vi "simulate or real stream sensorion data (subVI).vi"(0 "logfile refnum":refnum<file>, 1 "VISA resource name (COM3)":refnum<visa-resource-name>="COM3", 2 "stop channel":T2, 3 "abort? (F)":bool, 7 "simulate?":bool, 11 "error in (no error)":errorcluster) -> (4 "logfile refnum out":refnum<file>, 8 "sensor data cluster \nstream channel":T1, 15 "error out":errorcluster)   [LabVIEW 2021]
uses:
  <extravilib>/ChannelInstances/Tag-bool/))Channel.ctl
  <extravilib>/ChannelInstances/Stream-t'sensirion_data_with_time.ctl'/)Channel.ctl
  type-defs/sensirion_data_with_time.ctl
  controls/sensirion_flow_sensor_data.ctl
  <extravilib>/ChannelInstances/Tag-bool/Write With Abort.vi
  <extravilib>/ChannelInstances/Tag-bool/Read With Abort.vi
  <extravilib>/ChannelInstances/Stream-t'sensirion_data_with_time.ctl'/Read With Abort.vi
  <extravilib>/ChannelInstances/Stream-t'sensirion_data_with_time.ctl'/Write With Abort.vi
  <extravilib>/ChannelInstances/Stream-t'sensirion_data_with_time.ctl'/EndpointRead.vi
  <extravilib>/ChannelInstances/Stream-t'sensirion_data_with_time.ctl'/Endpoint.vi
  <extravilib>/ChannelInstances/Stream-t'sensirion_data_with_time.ctl'/Instantiate.vi
  <extravilib>/ChannelInstances/Tag-bool/Instantiate.vi
  <extravilib>/ChannelInstances/Tag-bool/Endpoint.vi
  <extravilib>/ChannelInstances/Tag-bool/EndpointRead.vi
  <extravilib>/ChannelInstances/Stream-t'sensirion_data_with_time.ctl'/)Channel.vi
  <resource>/ChannelSupport/_ChannelSupport/WaitIfNeeded.vi
  <extravilib>/ChannelInstances/Stream-t'sensirion_data_with_time.ctl'.lvlib
  <extravilib>/ChannelInstances/Tag-bool.lvlib
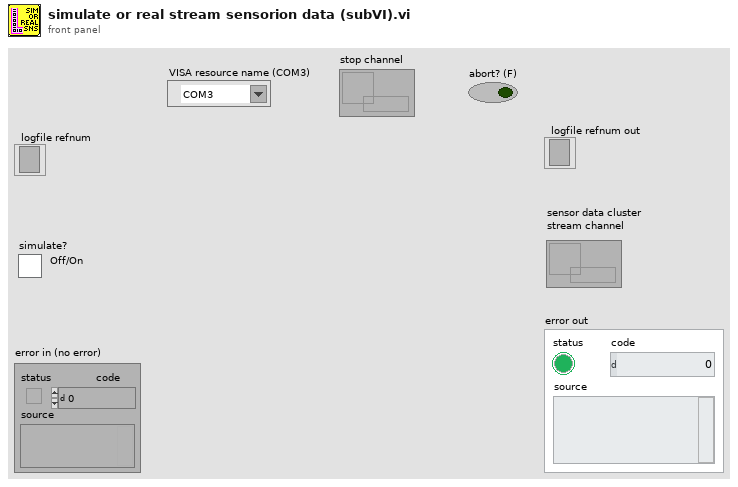
[diagram p1: front panel]
types:
  T1 = typedef "Stream-t'sensirion_data_with_time.ctl'.lvlib/)Channel.ctl" = refnum<queue>
  T2 = typedef "Tag-bool.lvlib/))Channel.ctl" = refnum<queue>
  T3 = typedef "sensirion_data_with_time.ctl" = cluster{"sensor data array":T4[], "relative timestamp":dbl, "error":errorcluster}
  T4 = typedef "sensirion_flow_sensor_data.ctl" = cluster{"flow rate \n":dbl[unit], "flow val. status":bool, "temperature":dbl[unit], "temp. val status":bool, "air in line?":bool, "high flow?":bool, "flag. val status":bool}
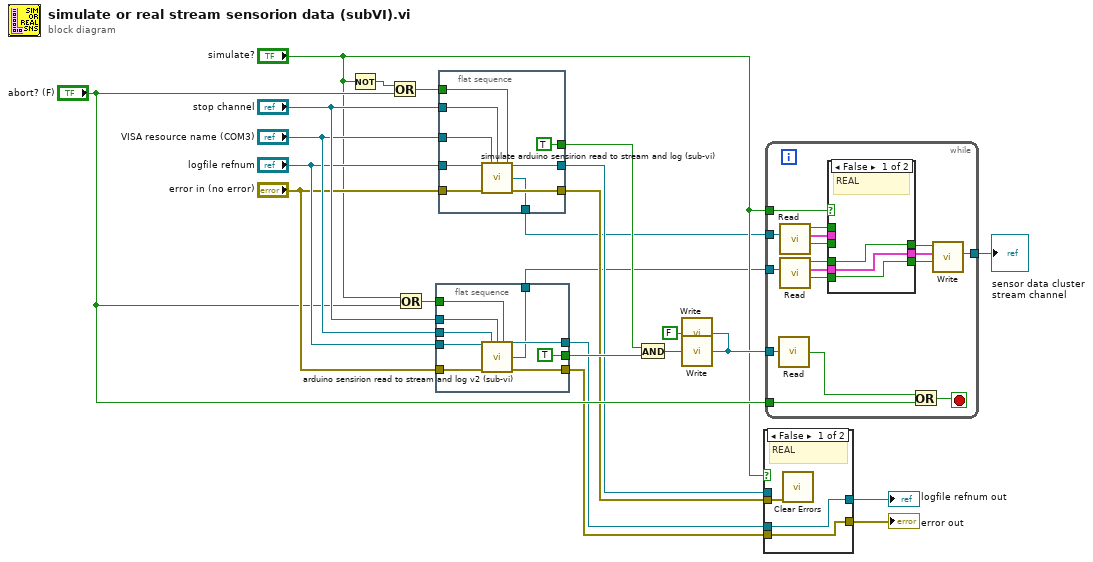
[diagram p0: block diagram]
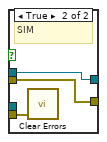
[diagram p2: hidden frame]
diagram:
  n1 = Not(x="simulate?") -> (.not. x?=w11:bool)
  n2 = Or(x=w11, y="abort? (F)") -> (x .or. y?=w19:bool)
  n3 = Or(x="simulate?", y="abort? (F)") -> (x .or. y?=w18:bool)
  n4 = flat-sequence {
    tunnel: [w24] -> w1
    tunnel: "stop channel" -> [w32]
    tunnel: "VISA resource name (COM3)" -> [w31]
    tunnel: "logfile refnum" -> [w30]
    tunnel: "error in (no error)" -> [w29]
    tunnel: w18 -> [w28]
    tunnel: [TRUE] -> w15
    tunnel: [w26] -> w5
    tunnel: [w25] -> w6
    frame #0 {
      n5 = call "arduino sensirion read to stream and log v2 (sub-vi).vi"("logfile refnum"=w30, "VISA resource name (COM3)"=w31, "stop? tag channel"=w32, "abort? (F)"=w28, "error in (no error)"=w29) -> ("logfile refnum out"=w25:refnum<file>, "sensor data cluster\nstream channel"=w24:T1, "error out"=w26:errorcluster)  [unwired: 8 in]
    }
  }
  n6 = flat-sequence {
    tunnel: "stop channel" -> [w41]
    tunnel: "VISA resource name (COM3)" -> [w40]
    tunnel: "logfile refnum" -> [w39]
    tunnel: "error in (no error)" -> [w38]
    tunnel: w19 -> [w37]
    tunnel: [w33] -> w2
    tunnel: [w36] -> w8
    tunnel: [w35] -> w7
    tunnel: [TRUE] -> w10
    frame #0 {
      n7 = call "simulate arduino sensirion read to stream and log (sub-vi).vi"("logfile refnum"=w39, "VISA resource name (COM3)"=w40, "stop channel"=w41, "abort? (F)"=w37, "error in (no error)"=w38) -> ("logfile refnum out"=w35:refnum<file>, "sensor data cluster channel"=w33:T1, "error out"=w36:errorcluster)  [unwired: 8 in]
    }
  }
  n8 = And(x=w10, y=w15) -> (x .and. y?=w14:bool)
  n9 = call <extravilib>:"Write.vi"("element"=FALSE) -> ("channel"=w12:T2)  [unwired: 1 out]
  n10 = call <extravilib>:"Write.vi"("element"=w14, "channel"=w12) -> ()  [unwired: 1 out]
  n11 = case shown="False" "simulate?" {
    tunnel: w8 -> [w42 w47]
    tunnel: w7 -> [_ w46]
    tunnel: w6 -> [w43 _]
    tunnel: w5 -> [w44 w45]
    tunnel: [w44 w47] -> w4
    tunnel: [w43 w46] -> w3
    frame False {
      # "REAL"
      n12 = call <vilib>:"Clear Errors.vi"("error in (no error)"=w42) -> ()  [unwired: 5 in, 2 out]
    }
    frame True {
      # "SIM"
      n13 = call <vilib>:"Clear Errors.vi"("error in (no error)"=w45) -> ()  [unwired: 5 in, 2 out]
    }
  }
  "error out" <- w4
  "logfile refnum out" <- w3
  n14 = while {
    tunnel: w2 -> [w64]
    tunnel: w1 -> [w63]
    tunnel: "simulate?" -> [w60]
    tunnel: [w55] -> w17
    tunnel: "abort? (F)" -> [w53]
    tunnel: w12 -> [w52]
    stop <- w54 stop-if-true
    n15 = call <extravilib>:"Read.vi"("channel"=w52) -> ("element"=w51:bool)  [unwired: 1 in, 1 out]
    n16 = call <extravilib>:"Read.vi"("channel"=w64) -> ("last element?"=w49:bool, "element"=w61:T3, "element valid?"=w59:bool)  [unwired: 6 in, 2 out]
    n17 = call <extravilib>:"Read.vi"("channel"=w63) -> ("last element?"=w50:bool, "element"=w62:T3, "element valid?"=w58:bool)  [unwired: 6 in, 2 out]
    n18 = case shown="False" w60 {
      tunnel: w62 -> [w66 _]
      tunnel: w61 -> [_ w69]
      tunnel: w59 -> [_ w70]
      tunnel: w58 -> [w67 _]
      tunnel: [w67 w70] -> w56
      tunnel: [w66 w69] -> w57
      tunnel: w50 -> [w65 _]
      tunnel: w49 -> [_ w68]
      tunnel: [w65 w68] -> w48
      frame False {
        # "REAL"
      }
      frame True {
        # "SIM."
      }
    }
    n19 = Or(x=w51, y=w53) -> (x .or. y?=w54:bool)
    n20 = call <extravilib>:"Write.vi"("last element? (F)"=w48, "element"=w57, "element valid? (T)"=w56) -> ("channel"=w55:T1)  [unwired: 6 in, 2 out]
  }
  "sensor data cluster \nstream channel" <- w17
